vi "FITS_WriteKeyFromChar.vi"(0 "ref":u64, 5 "datatype":i32, 7 "keyname":string, 9 "value":string, 11 "error in (no error)":errorcluster, 12 "comment":string) -> (4 "keyname out":string, 6 "value out":string, 8 "comment out":string, 10 "return type":i32, 15 "error out":errorcluster)   [LabVIEW 2016]
uses:
  usr/local/lib/libfits.so
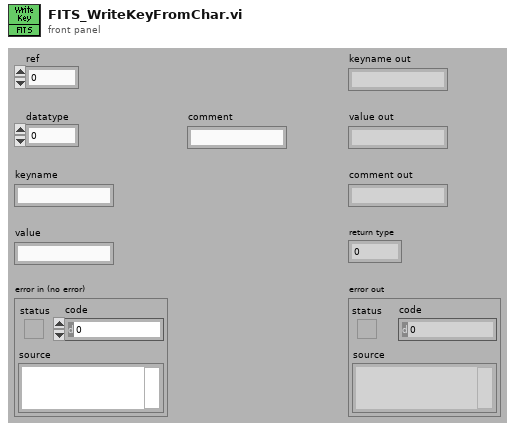
[diagram p1: front panel]
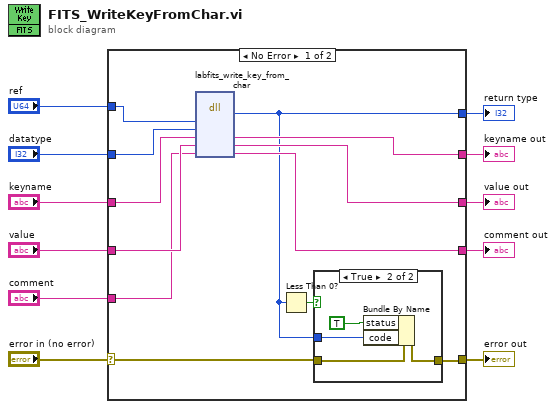
[diagram p0: block diagram]
diagram:
  n1 = case shown="No Error" "error in (no error)" {
    selector: "error in (no error)" -> [w14 w32]
    tunnel: [w13 w32] -> w10
    tunnel: [w12 _] -> w9
    tunnel: "ref" -> [w23 _]
    tunnel: "datatype" -> [w22 _]
    tunnel: "keyname" -> [w21 w31]
    tunnel: [w20 w31] -> w5
    tunnel: "value" -> [w19 w30]
    tunnel: [w18 w30] -> w3
    tunnel: "comment" -> [w17 w29]
    tunnel: [w16 w29] -> w1
    frame No Error {
      n2 = dll-call lib="usr/local/lib/libfits.so" fn="labfits_write_key_from_char"("ref"=w23, "datatype"=w22, "keyname"=w21, "value"=w19, "comment"=w17) -> ("return type"=w12:i32, "keyname"=w20:string, "value"=w18:string, "comment"=w16:string)  [unwired: 5 in, 2 out]
      n3 = Less Than 0?(x=w12) -> (x < 0?=w15:bool)
      n4 = case shown="True" w15 {
        tunnel: w14 -> [w24 w26]
        tunnel: [w24 w25] -> w13
        tunnel: w12 -> [_ w27]
        frame False {
        }
        frame True {
          n5 = Bundle By Name(cluster=w26, "status"=TRUE, "code"=w27) -> (w25:errorcluster)
        }
      }
    }
    frame Error {
    }
  }
  "return type" <- w9
  "keyname out" <- w5
  "value out" <- w3
  "comment out" <- w1
  "error out" <- w10
